vi "Global 1.vi"() -> ()   [LabVIEW 2020, in "GetSetShared.lvlib"]
uses:
  <vilib>/express/express signal manip/GetorSetDDTAttributes/Shared VIs/GetSetShared.lvlib
  <vilib>/BlockNodeSupport/TerminalData.ctl
panel:
  in  "Get DDT.Instance VI Name":string="Get Dynamic Data Attributes"
  in  "Set DDT.Instance VI Name":string="Set Dynamic Data Attributes"
  in  "error message":string="Error occurs when loading the Express VI."
  in  "Terminal ID":string[](array[string])=["Signals In", "Signals Out", "error in", "error out", "Signal Index"]
  in  "Set.Terminal Data 2":T1[](array[typedef])=[{"Terminal Name"="Signals In", "Terminal Display Name"="Signals In", "Terminal ID"="Signals In", "Terminal Flags"=517, "Terminal Type"=variant(dynamicdata []), "Terminal Map ID"=0}, {"Terminal Name"="Signals Out", "Terminal Display Name"="Signals Out", "Terminal ID"="Signals Out", "Terminal Flags"=525, "Terminal Type"=variant(dynamicdata []), "Terminal Map ID"=4}, {"Terminal Name"="error in", "Terminal Display Name"="error in", "Terminal ID"="error in", "Terminal Flags"=513, "Terminal Type"=variant(errorcluster {"status"=FALSE, "code"=0, "source"=""}), "Terminal Map ID"=11}, {"Terminal Name"="error out", "Terminal Display Name"="error out", "Terminal ID"="error out", "Terminal Flags"=521, "Terminal Type"=variant(errorcluster {"status"=FALSE, "code"=0, "source"=""}), "Terminal Map ID"=15}, {"Terminal Name"="Signal Index", "Terminal Display Name"="Signal Index", "Terminal ID"="Signal Index", "Terminal Flags"=517, "Terminal Type"=variant(i32 0), "Terminal Map ID"=5}, {"Terminal Name"="Signal Name", "Terminal Display Name"="Signal Name", "Terminal ID"="Signal Name", "Terminal Flags"=513, "Terminal Type"=variant(string ""), "Terminal Map ID"=6}, {"Terminal Name"="Time Mode", "Terminal Display Name"="Time Mode", "Terminal ID"="Time Mode", "Terminal Flags"=513, "Terminal Type"=variant(enum16{"Absolute", "Relative"} enum."Absolute"), "Terminal Map ID"=8}, {"Terminal Name"="Timestamp", "Terminal Display Name"="Timestamp", "Terminal ID"="Timestamp", "Terminal Flags"=513, "Terminal Type"=variant(timestamp timestamp(0 s since 1904-01-01)), "Terminal Map ID"=10}, {"Terminal Name"="Start Timestamp", "Terminal Display Name"="Start Timestamp", "Terminal ID"="Start Timestamp", "Terminal Flags"=513, "Terminal Type"=variant(timestamp timestamp(0 s since 1904-01-01)), "Terminal Map ID"=3}, {"Terminal Name"="X Dimension", "Terminal Display Name"="X Dimension", "Terminal ID"="X Dimension", "Terminal Flags"=513, "Terminal Type"=variant(enum16{"No Unit [-]", "Time [sec]", "Frequency [Hz]"} enum."No Unit [-]"), "Terminal Map ID"=2}, {"Terminal Name"="Unit", "Terminal Display Name"="Unit", "Terminal ID"="Unit", "Terminal Flags"=513, "Terminal Type"=variant(string ""), "Terminal Map ID"=14}] {"Terminal Flags" format="%.0b"}
  in  "Set.Terminal Data":T1[](array[typedef])=[{"Terminal Name"="Signals In", "Terminal Display Name"="Signals In", "Terminal ID"="Signals In", "Terminal Flags"=517, "Terminal Type"=variant(dynamicdata []), "Terminal Map ID"=0}, {"Terminal Name"="Signals Out", "Terminal Display Name"="Signals Out", "Terminal ID"="Signals Out", "Terminal Flags"=525, "Terminal Type"=variant(dynamicdata []), "Terminal Map ID"=4}, {"Terminal Name"="error in", "Terminal Display Name"="error in", "Terminal ID"="error in", "Terminal Flags"=513, "Terminal Type"=variant(errorcluster {"status"=FALSE, "code"=0, "source"=""}), "Terminal Map ID"=11}, {"Terminal Name"="error out", "Terminal Display Name"="error out", "Terminal ID"="error out", "Terminal Flags"=521, "Terminal Type"=variant(errorcluster {"status"=FALSE, "code"=0, "source"=""}), "Terminal Map ID"=15}, {"Terminal Name"="Signal Index", "Terminal Display Name"="Signal Index", "Terminal ID"="Signal Index", "Terminal Flags"=517, "Terminal Type"=variant(i32 0), "Terminal Map ID"=5}] {"Terminal Flags" format="%.0b"}
  in  "Get.Terminal Data":T1[](array[typedef])=[{"Terminal Name"="Signals In", "Terminal Display Name"="Signals In", "Terminal ID"="Signals In", "Terminal Flags"=517, "Terminal Type"=variant(dynamicdata []), "Terminal Map ID"=0}, {"Terminal Name"="Signals Out", "Terminal Display Name"="Signals Out", "Terminal ID"="Signals Out", "Terminal Flags"=521, "Terminal Type"=variant(dynamicdata []), "Terminal Map ID"=4}, {"Terminal Name"="error in", "Terminal Display Name"="error in", "Terminal ID"="error in", "Terminal Flags"=513, "Terminal Type"=variant(errorcluster {"status"=FALSE, "code"=0, "source"=""}), "Terminal Map ID"=11}, {"Terminal Name"="error out", "Terminal Display Name"="error out", "Terminal ID"="error out", "Terminal Flags"=521, "Terminal Type"=variant(errorcluster {"status"=FALSE, "code"=0, "source"=""}), "Terminal Map ID"=15}, {"Terminal Name"="Signal Index", "Terminal Display Name"="Signal Index", "Terminal ID"="Signal Index", "Terminal Flags"=517, "Terminal Type"=variant(i32 0), "Terminal Map ID"=5}] {"Terminal Flags" format="%.0b"}
  in  "TermSignalName":string="Signal Name"
  in  "TermUnit":string="Unit"
  in  "TermXDimension":string="X Dimension"
  in  "TermStartTimeStamp":string="Start Timestamp"
  in  "TermTimeStamp":string="Timestamp"
  in  "TermTimeMode":string="Time Mode"
  in  "TermErrorIn":string="error in"
  in  "TermErrorOut":string="error out"
  in  "TermSignalsOut":string="Signals Out"
  in  "TermSignalIndex":string="Signal Index"
  in  "TermSignalsIn":string="Signals In"
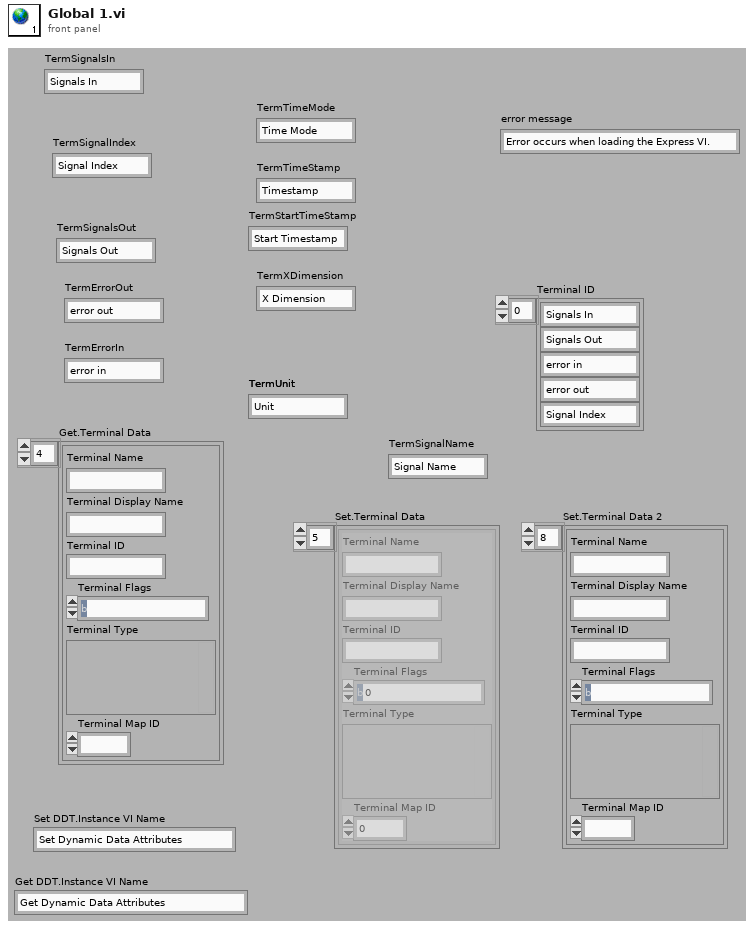
[diagram p1: front panel]
types:
  T1 = typedef "TerminalData.ctl" = cluster{"Terminal Name":string, "Terminal Display Name":string, "Terminal ID":string, "Terminal Flags":i32, "Terminal Type":variant, "Terminal Map ID":i32}
diagram:
